vi "readComCommandt.vi"() -> ()   [LabVIEW 2016]
uses:
  ElectrometerConfiguration/Controls/com_conf.ctl
  ts_electrometeruserevents/Typedefs/termChar.ctl
  Electrometer/Electrometer.lvclass
  ElectrometerConfiguration/ElectrometerCOMConfiguration.lvclass
  ts_electrometeruserevents/Typedefs/ElectrometerTypedefs.lvlib
  ts_electrometeruserevents/ConfigurationTC/ConfigurationTypedefs/ConfigurationTypedefs.lvlib
panel:
  out "x-y":dbl
  out "read buffer 4":string
  out "read buffer 3":string
  in  "Fix":bool
  out "read buffer 2":string
  in  "saveFiles":bool
  in  "sendCMD":bool
  out "read buffer":string
  in  "string":string=":TRAC:POIN:ACT? "
  out "error out disccnect":errorcluster
  in  "sendQuery":bool
  in  "stop":bool
  in  "Serial Communication":T1={"Baud Rate"=57600.0, "VISA resource name"="ASRL5::INSTR", "Parity"=0, "Data Bits"=8, "Stop Bits"=10, "Flow Control"=0, "termChar"=enum."LF"} {"Flow Control" items=["None", "XON/XOFF", "RTS/CTS", "XON/XOFF & RTS/CTS", "DTR/DSR", "XON/XOFF & DTR/DSR"]; "Stop Bits" items=["1.0"=10, "1.5"=15, "2.0"=20]; "Data Bits" items=["7"=7, "8"=8]; "Parity" items=["None", "Odd", "Even", "Mark", "Space"]}
  out "Error Message":string
  out "Error Code":i32[](array[numeric])
  out "error out":errorcluster
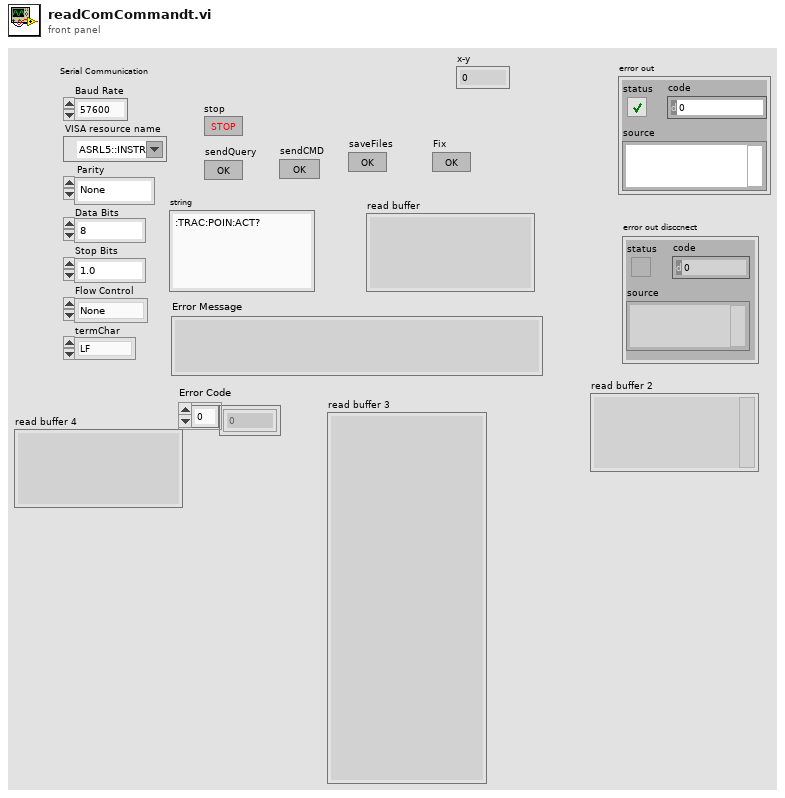
[diagram p1: front panel]
types:
  T1 = typedef "ConfigurationTypedefs.lvlib/com_conf.ctl" = cluster{"Baud Rate":dbl, "VISA resource name":refnum<visa-resource-name>, "Parity":u16, "Data Bits":u16, "Stop Bits":u16, "Flow Control":u16, "termChar":T2}
  T2 = typedef "ElectrometerTypedefs.lvlib/termChar.ctl" = enum16{"CR", "CR+LF", "LF", "LF+CR"}
  T3 = enum16{"open", "replace", "create", "open or create", "replace or create", "replace or create with confirmation"}
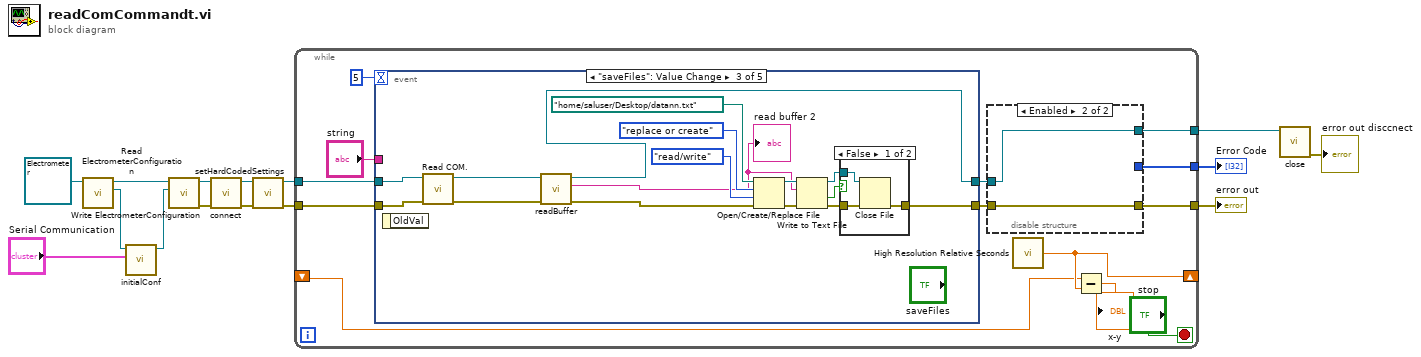
[diagram p0: block diagram]
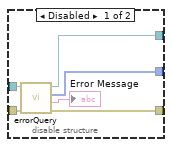
[diagram p2: hidden frame]
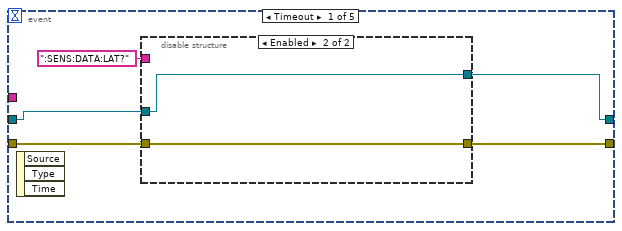
[diagram p3: hidden frame]
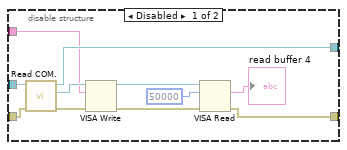
[diagram p4: hidden frame]
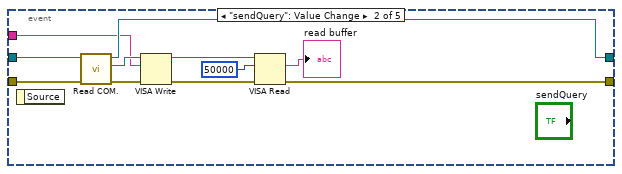
[diagram p5: hidden frame]
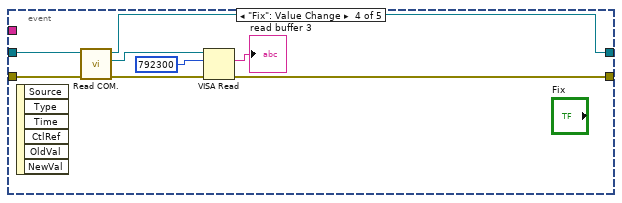
[diagram p7: hidden frame]
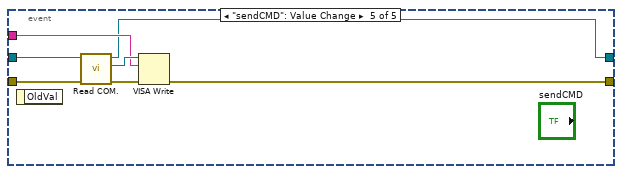
[diagram p8: hidden frame]
diagram:
  n1 = call "Read ElectrometerConfiguration.vi"("Electrometer in"=refnum<class "Electrometer.lvclass"> refnum ("Electrometer.lvclass")) -> ("ElectrometerConfiguration"=w13:refnum<class "ElectrometerCOMConfiguration.lvclass">, "Electrometer out"=w14:refnum<class "Electrometer.lvclass">)  [unwired: 8 in, 1 out]
  n2 = call "initialConf.vi"("Serial Communication"="Serial Communication", "ElectrometerConfiguration In"=w13) -> ("ElectrometerConfiguration Out"=w12:refnum<class "ElectrometerCOMConfiguration.lvclass">)  [unwired: 9 in]
  n3 = call-dynamic "Write ElectrometerConfiguration.vi"("ElectrometerConfiguration"=w12, "Electrometer in"=w14) -> ("error out"=w10:errorcluster, "Electrometer out"=w11:refnum<class "Electrometer.lvclass">)  [unwired: 8 in]
  n4 = call "connect.vi"("error in (no error)"=w10, "Electrometer in"=w11) -> ("error out"=w4:errorcluster, "Electrometer out"=w1:refnum<class "Electrometer.lvclass">)  [unwired: 7 in, 1 out]
  n5 = call "setHardCodedSettings.vi"("error in (no error)"=w4, "Electrometer in"=w1) -> ("error out"=w3:errorcluster, "Electrometer out"=w2:refnum<class "Electrometer.lvclass">)  [unwired: 8 in]
  n6 = while {
    tunnel: [w28] -> w9
    tunnel: [w27] -> w6
    tunnel: w3 -> [w23]
    tunnel: [w25] -> w7
    tunnel: w2 -> [w24]
    shift-right: [w18] -> _
    shift-left: _ -> [w17]
    stop <- "stop" stop-if-true
    n7 = event shown="[2] \"saveFiles\": Value Change" {
      selector: _ -> [_ _ _ _ _]
      dyn-events: _ -> [_ _ _ _ _]
      timeout: 5 -> [_ _ _ _ _]
      tunnel: w24 -> [w41 w60 w81 w91 w97]
      tunnel: w23 -> [w40 w59 w80 w92 w96]
      tunnel: [w39 w58 w77 w87 w94] -> w22
      tunnel: [w38 w57 w69 w90 w95] -> w21
      tunnel: "string" -> [_ w56 _ _ w98]
      event Timeout {
        n8 = event-data() -> ()  [unwired: 1 in, 3 out]
        n9 = disable-structure shown="Enabled" {
          disable-tunnel: w41 -> [w46 w54]
          disable-tunnel: w40 -> [w45 w53]
          disable-tunnel: [w44 w53] -> w39
          disable-tunnel: [w43 w54] -> w38
          disable-tunnel: ":SENS:DATA:LAT?" ("write buffer") -> [w42 _]
          frame Disabled {
            n10 = call "Read COM..vi"("error in (no error)"=w45, "Electrometer in"=w46) -> ("error out"=w51:errorcluster, "VISA"=w52:refnum<visa-resource-name>, "Electrometer out"=w43:refnum<class "Electrometer.lvclass">)  [unwired: 7 in]
            n11 = VISA Write(VISA resource name=w52, write buffer=w42, error in (no error)=w51) -> (VISA resource name out=w49:refnum<visa-resource-name>, error out=w50:errorcluster)  [unwired: 1 out]
            n12 = VISA Read(VISA resource name=w49, byte count=u32 50000, error in (no error)=w50) -> (read buffer=→"read buffer 4":string, error out=w44:errorcluster)  [unwired: 2 out]
          }
          frame Enabled {
          }
        }
      }
      event "sendQuery": Value Change {
        n13 = event-data() -> ()  [unwired: 1 in, 1 out]
        n14 = call "Read COM..vi"("error in (no error)"=w59, "Electrometer in"=w60) -> ("error out"=w64:errorcluster, "VISA"=w65:refnum<visa-resource-name>, "Electrometer out"=w57:refnum<class "Electrometer.lvclass">)  [unwired: 7 in]
        n15 = VISA Write(VISA resource name=w65, write buffer=w56, error in (no error)=w64) -> (VISA resource name out=w62:refnum<visa-resource-name>, error out=w63:errorcluster)  [unwired: 1 out]
        n16 = VISA Read(VISA resource name=w62, byte count=u32 50000, error in (no error)=w63) -> (read buffer=→"read buffer":string, error out=w58:errorcluster)  [unwired: 2 out]
      }
      event "saveFiles": Value Change {
        n17 = event-data() -> ()  [unwired: 1 in, 1 out]
        n18 = call "Read COM..vi"("error in (no error)"=w80, "Electrometer in"=w81) -> ("error out"=w66:errorcluster, "Electrometer out"=w70:refnum<class "Electrometer.lvclass">)  [unwired: 7 in, 1 out]
        n19 = call "readBuffer.vi"("error in (no error)"=w66, "Electrometer in"=w70) -> ("error out"=w67:errorcluster, "data"=w68:string, "Electrometer out"=w69:refnum<class "Electrometer.lvclass">)  [unwired: 7 in]
        "read buffer 2" <- w68
        n20 = Open/Create/Replace File(file path (use dialog)=path "/home/saluser/Desktop/datann.txt" ("file (use dialog)"), error in=w67, operation (0:open)=T3."replace or create", access (0:read/write)=enum16{"read/write", "read-only", "write-only"}."read/write") -> (refnum out=w71:refnum<file>, error out=w72:errorcluster)  [unwired: 2 in, 1 out]
        n21 = Write to Text File(file (use dialog)=w71, text=w68, error in=w72) -> (refnum out=w78:refnum<file>, cancelled=w76:bool, error out=w79:errorcluster)  [unwired: 1 in]
        n22 = case shown="False" w76 {
          tunnel: w79 -> [w84 w85]
          tunnel: w78 -> [w83 _]
          tunnel: [w82 w85] -> w77
          frame False {
            n23 = Close File(refnum=w83, error in=w84) -> (error out=w82:errorcluster)  [unwired: 1 out]
          }
          frame True {
          }
        }
      }
      event "Fix": Value Change {
        n24 = event-data() -> ()  [unwired: 1 in, 6 out]
        n25 = call "Read COM..vi"("error in (no error)"=w92, "Electrometer in"=w91) -> ("error out"=w88:errorcluster, "VISA"=w89:refnum<visa-resource-name>, "Electrometer out"=w90:refnum<class "Electrometer.lvclass">)  [unwired: 7 in]
        n26 = VISA Read(VISA resource name=w89, byte count=u32 792300, error in (no error)=w88) -> (read buffer=→"read buffer 3":string, error out=w87:errorcluster)  [unwired: 2 out]
      }
      event "sendCMD": Value Change {
        n27 = event-data() -> ()  [unwired: 1 in, 1 out]
        n28 = call "Read COM..vi"("error in (no error)"=w96, "Electrometer in"=w97) -> ("error out"=w99:errorcluster, "VISA"=w100:refnum<visa-resource-name>, "Electrometer out"=w95:refnum<class "Electrometer.lvclass">)  [unwired: 7 in]
        n29 = VISA Write(VISA resource name=w100, write buffer=w98, error in (no error)=w99) -> (error out=w94:errorcluster)  [unwired: 2 out]
      }
    }
    n30 = disable-structure shown="Enabled" {
      disable-tunnel: [w34 _] -> w28
      disable-tunnel: [w33 w35] -> w27
      disable-tunnel: [w32 w36] -> w25
      disable-tunnel: w22 -> [w31 w35]
      disable-tunnel: w21 -> [w30 w36]
      frame Disabled {
        n31 = call "errorQuery.vi"("error in (no error)"=w31, "Electrometer in"=w30) -> ("error out"=w33:errorcluster, "Error Message"=→"Error Message":string, "Device Error"=w34:i32[], "Electrometer out"=w32:refnum<class "Electrometer.lvclass">)  [unwired: 6 in]
      }
      frame Enabled {
      }
    }
    n32 = call <vilib>:"High Resolution Relative Seconds.vi"() -> ("relative seconds"=w18:dbl)
    n33 = Subtract(x=w17, y=w18) -> (x-y=→"x-y":dbl)
  }
  "error out" <- w6
  "Error Code" <- w9
  n34 = call "close.vi"("Electrometer in"=w7) -> ("error out"=→"error out disccnect":errorcluster)  [unwired: 9 in, 1 out]
